vi "X Range Change User Event.vi"(7 "All":bool, 8 "error in (no error)":errorcluster, 9 "Upper Range":dbl, 10 "Lower Range":dbl, 11 "XYGraphOverview in":refnum<class "XYGraphOverview.lvclass">) -> (0 "error out":errorcluster, 3 "XYGraphOverview out":refnum<class "XYGraphOverview.lvclass">)   [LabVIEW 2020, in "XYGraphOverview.lvlib" / "XYGraphOverview.lvclass"]
uses:
  XYGraphOverview.lvclass
  X Range Change User Event Data.ctl
  XYGraphOverview.lvclass/XYGraphOverview.ctl
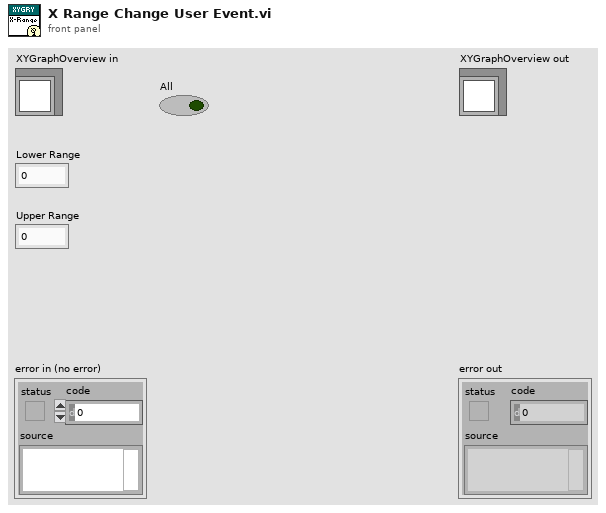
[diagram p1: front panel]
types:
  T1 = typedef "XYGraphOverview.lvlib/XYGraphOverview.lvclass/X Range Change User Event Data.ctl" = cluster{"Lower Range":dbl, "Upper Range":dbl, "All":bool}
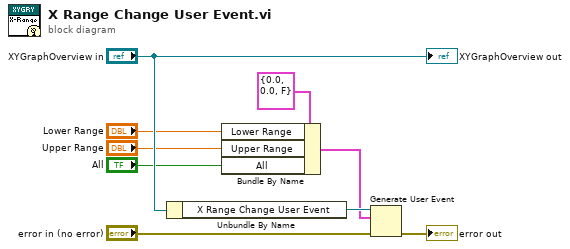
[diagram p0: block diagram]
diagram:
  n1 = Unbundle By Name("XYGraphOverview in") -> ("X Range Change User Event"=w6:refnum<user-event>)
  n2 = Bundle By Name(cluster=T1 {"Lower Range"=0.0, "Upper Range"=0.0, "All"=FALSE} ("event data"), "Lower Range"="Lower Range", "Upper Range"="Upper Range", "All"="All") -> (w4:T1)
  n3 = Generate User Event(user event=w6, event data cluster=w4, error in="error in (no error)") -> (error out=→"error out":errorcluster)  [unwired: 1 in, 1 out]
  "XYGraphOverview out" <- "XYGraphOverview in"
